vi "ConfigureGroups.vi"(6 "all channels":T1[](array[typedef]), 8 "error in (no error)":errorcluster, 10 "acquisition channels (in acquisition order)":T1[](array[typedef]), 11 "device":T4) -> (0 "error out":errorcluster, 3 "groups":T11[](array[typedef]))   [LabVIEW 2017, in "CmsAcquisition.lvlib"]
uses:
  <vilib>/addons/InsightCM/Devices/Shared/Cms/CmsAcquisition/CmsAcquisition.lvlib
  <vilib>/addons/InsightCM/MessageBus/Base/controls/R2_Channel.ctl
  <vilib>/addons/InsightCM/MessageBus/Base/controls/KeyValuePair.ctl
  <vilib>/addons/InsightCM/MessageBus/Base/controls/Metric.ctl
  <vilib>/addons/InsightCM/Devices/Shared/Cms/CmsAcquisition/controls/Group.ctl
  <vilib>/addons/InsightCM/Devices/Shared/Cms/CmsAcquisition/controls/Channel.ctl
  <vilib>/addons/InsightCM/MessageBus/Base/controls/R2_Device.ctl
  <vilib>/addons/InsightCM/MessageBus/Base/controls/DeviceState.ctl
  <vilib>/addons/InsightCM/MessageBus/Base/controls/R2_DataGroup.ctl
  <vilib>/addons/InsightCM/MessageBus/Base/controls/OperatingState.ctl
  <vilib>/addons/InsightCM/MessageBus/Base/controls/Trigger.ctl
  <vilib>/addons/InsightCM/MessageBus/Base/controls/Condition.ctl
  <vilib>/addons/InsightCM/MessageBus/Base/controls/BurstModeTrigger.ctl
  <vilib>/addons/InsightCM/MessageBus/Base/controls/R2_DeviceModel.ctl
  <vilib>/addons/InsightCM/MessageBus/Base/controls/Tag.ctl
  <vilib>/addons/InsightCM/Utilities/DeviceModelHelpers/DeviceModelHelpers.lvlib
  <vilib>/addons/InsightCM/Utilities/PropertyHelpers/PropertyHelpers.lvlib
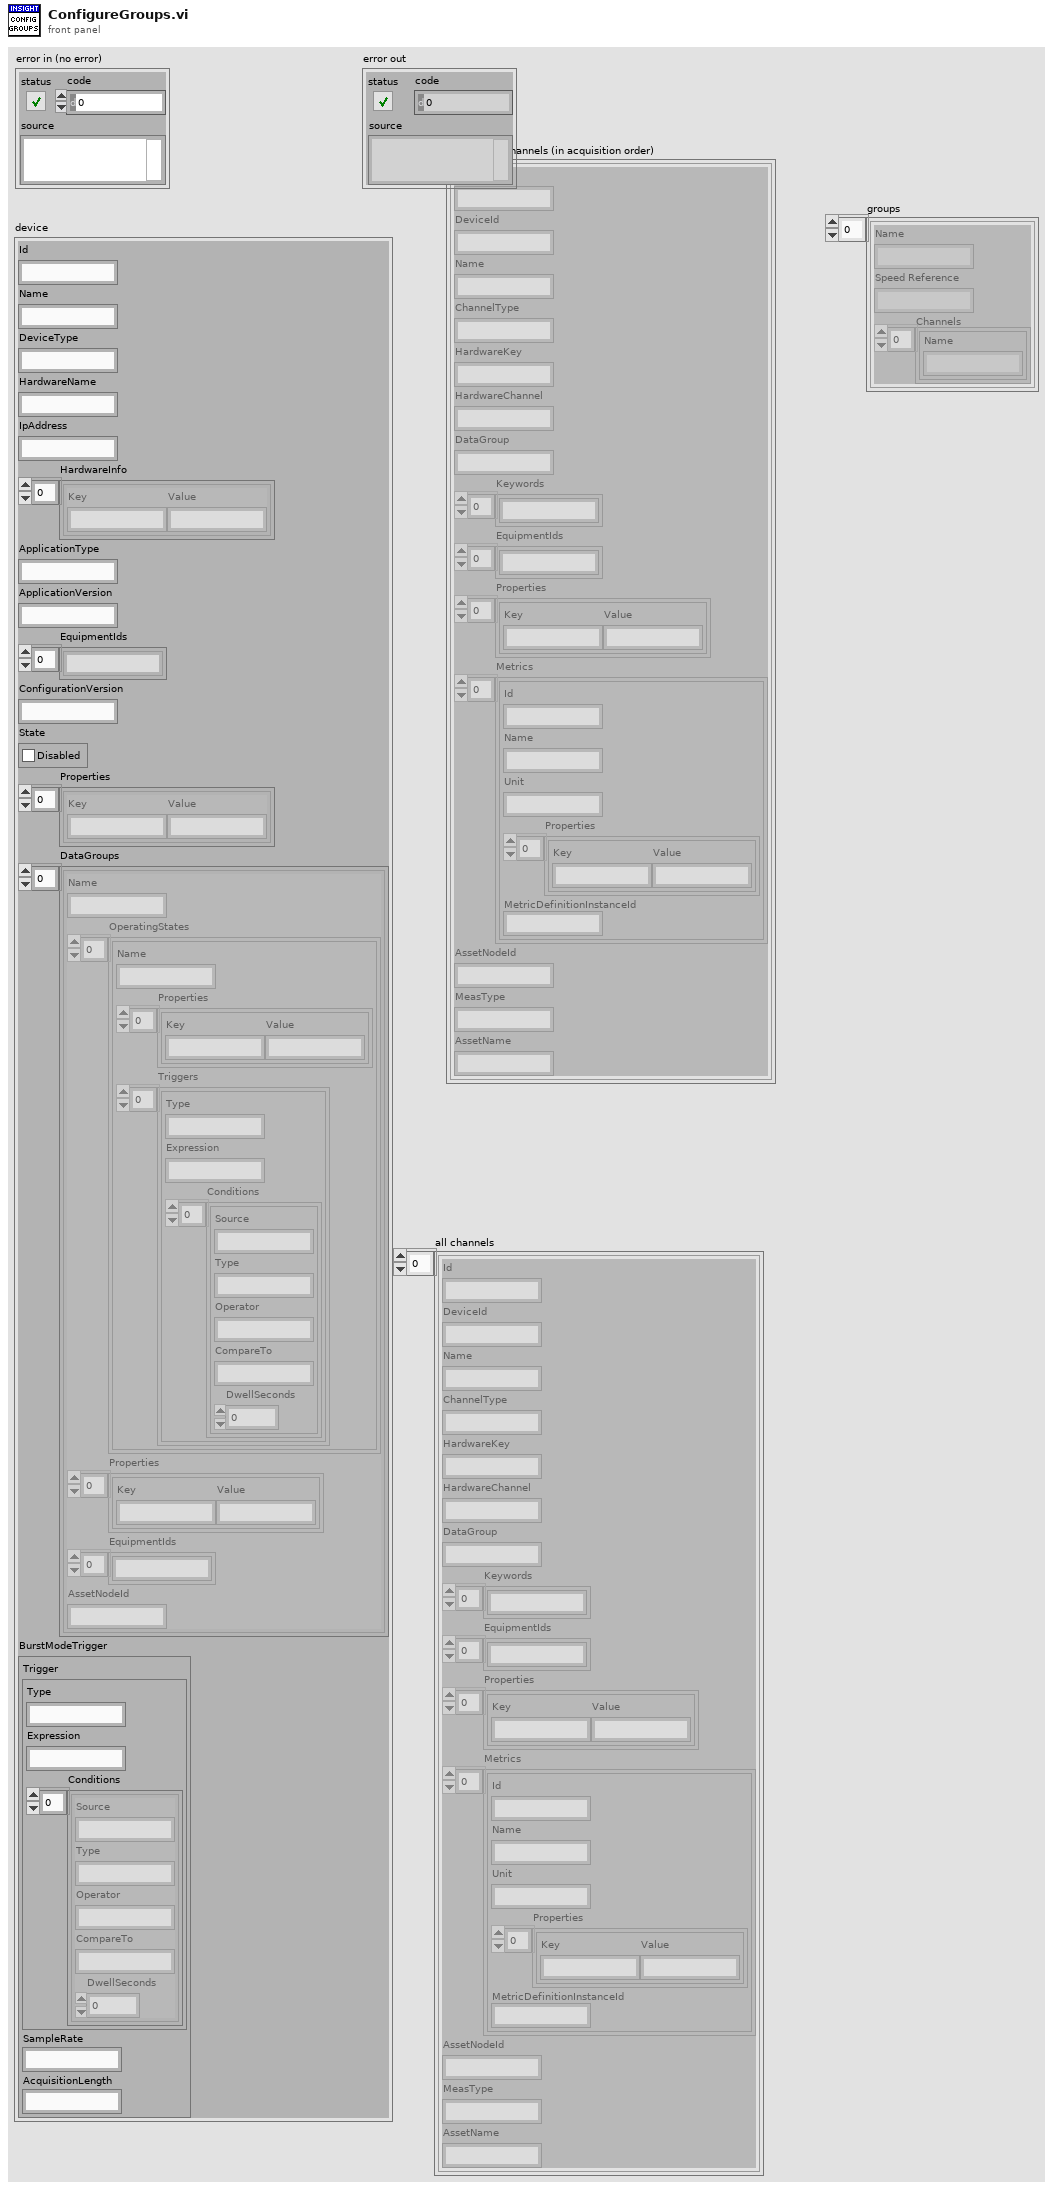
[diagram p1: front panel]
types:
  T1 = typedef "R2_Channel.ctl" = cluster{"Id":string, "DeviceId":string, "Name":string, "ChannelType":string, "HardwareKey":string, "HardwareChannel":string, "DataGroup":string, "Keywords":string[], "EquipmentIds":string[], "Properties":T2[], "Metrics":T3[], "AssetNodeId":string, "MeasType":string, "AssetName":string}
  T2 = typedef "KeyValuePair.ctl" = cluster{"Key":string, "Value":string}
  T3 = typedef "Metric.ctl" = cluster{"Id":string, "Name":string, "Unit":string, "Properties":T2[], "MetricDefinitionInstanceId":string}
  T4 = typedef "R2_Device.ctl" = cluster{"Id":string, "Name":string, "DeviceType":string, "HardwareName":string, "IpAddress":string, "HardwareInfo":T2[], "ApplicationType":string, "ApplicationVersion":string, "EquipmentIds":string[], "ConfigurationVersion":string, "State":T5, "Properties":T2[], "DataGroups":T6[], "BurstModeTrigger":T10}
  T5 = typedef "DeviceState.ctl" = cluster{"Disabled":bool}
  T6 = typedef "R2_DataGroup.ctl" = cluster{"Name":string, "OperatingStates":T7[], "Properties":T2[], "EquipmentIds":string[], "AssetNodeId":string}
  T7 = typedef "OperatingState.ctl" = cluster{"Name":string, "Properties":T2[], "Triggers":T8[]}
  T8 = typedef "Trigger.ctl" = cluster{"Type":string, "Expression":string, "Conditions":T9[]}
  T9 = typedef "Condition.ctl" = cluster{"Source":string, "Type":string, "Operator":string, "CompareTo":string, "DwellSeconds":dbl}
  T10 = typedef "BurstModeTrigger.ctl" = cluster{"Trigger":T8, "SampleRate":string, "AcquisitionLength":string}
  T11 = typedef "CmsAcquisition.lvlib/Group.ctl" = cluster{"Name":string, "Speed Reference":string, "Channels":T12[]}
  T12 = typedef "CmsAcquisition.lvlib/Channel.ctl" = cluster{"Name":string}
  T13 = typedef "R2_DeviceModel.ctl" = cluster{"Device":T4, "Channels":T1[], "Tags":T14[]}
  T14 = typedef "Tag.ctl" = cluster{"Id":string, "Path":string, "Name":string, "Datatype":string, "Props":T2[], "Keywords":string[]}
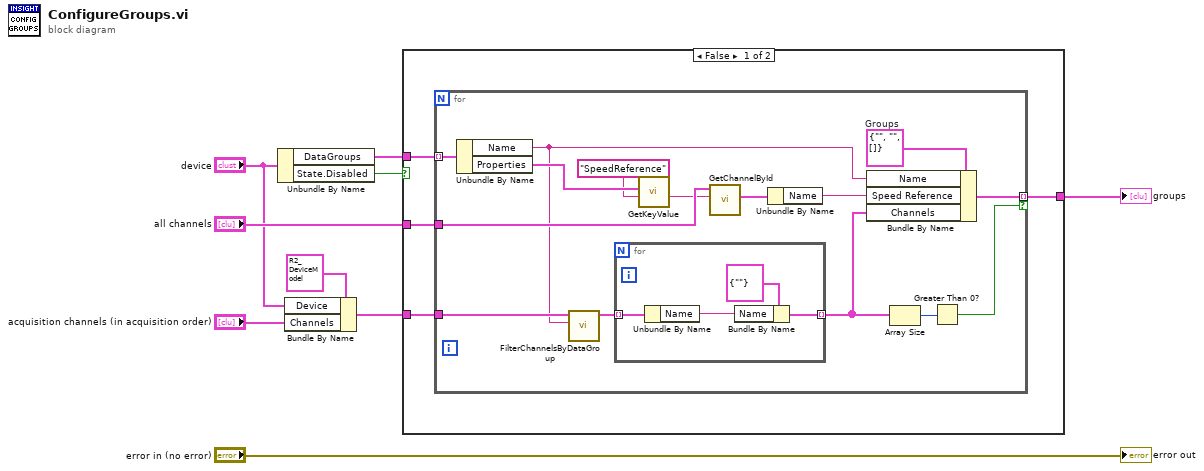
[diagram p0: block diagram]
diagram:
  n1 = Unbundle By Name("device") -> ("DataGroups"=w8:T6[], "State.Disabled"=w1:bool)
  n2 = Bundle By Name(cluster=T13 {"Device"={"Id"="", "Name"="", "DeviceType"="", "HardwareName"="", "IpAddress"="", "HardwareInfo"=[], "ApplicationType"="", "ApplicationVersion"="", "EquipmentIds"=[], "ConfigurationVersion"="", "State"={"Disabled"=FALSE}, "Properties"=[], "DataGroups"=[], "BurstModeTrigger"={"Trigger"={"Type"="", "Expression"="", "Conditions"=[]}, "SampleRate"="", "AcquisitionLength"=""}}, "Channels"=[], "Tags"=[]} ("device model"), "Device"="device", "Channels"="acquisition channels (in acquisition order)") -> (w5:T13)
  n3 = case shown="False" w1 {
    tunnel: [w13 _] -> w9
    tunnel: w8 -> [w12 _]
    tunnel: w5 -> [w11 _]
    tunnel: "all channels" -> [w10 _]
    frame False {
      n4 = for {
        tunnel: w12 -> [w28] mode=indexing
        tunnel: [w26] -> w13 mode=indexing if=w23
        tunnel: w11 -> [w22]
        tunnel: w10 -> [w20]
        w27 = T11 {"Name"="", "Speed Reference"="", "Channels"=[]}  # Groups
        n5 = Unbundle By Name(w28) -> ("Name"=w14:string, "Properties"=w17:T2[])
        n6 = call <vilib>:"FilterChannelsByDataGroup.vi"("group"=w14, "device model"=w22) -> ("channels in data group"=w21:T1[])  [unwired: 8 in, 1 out]
        n7 = for {
          tunnel: [w32] -> w25 mode=indexing
          tunnel: w21 -> [w31] mode=indexing
          n8 = Unbundle By Name(w31) -> ("Name"=w29:string)
          n9 = Bundle By Name(cluster=T12 {"Name"=""} ("channel"), "Name"=w29) -> (w32:T12)
        }
        n10 = call <vilib>:"GetKeyValue.vi"("key"="SpeedReference", "key value pairs"=w17) -> ("value"=w16:string)  [unwired: 7 in, 2 out]
        n11 = call <vilib>:"GetChannelById.vi"("channel id"=w16, "channels in"=w20) -> ("channel"=w19:T1)  [unwired: 7 in, 2 out]
        n12 = Unbundle By Name(w19) -> ("Name"=w18:string)
        n13 = Bundle By Name(cluster=w27, "Name"=w14, "Speed Reference"=w18, "Channels"=w25) -> (w26:T11)
        n14 = Array Size(array=w25) -> (size(s)=w24:i32)
        n15 = Greater Than 0?(x=w24) -> (x > 0?=w23:bool)
      }
    }
    frame True {
    }
  }
  "groups" <- w9
  "error out" <- "error in (no error)"
